vi "COM Stage Test Write.vi"() -> ()   [LabVIEW 2017]
panel:
  out "Numeric":i32
  in  "Position (mm)":dbl
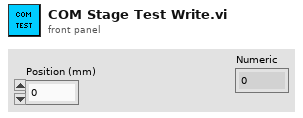
[diagram p1: front panel]
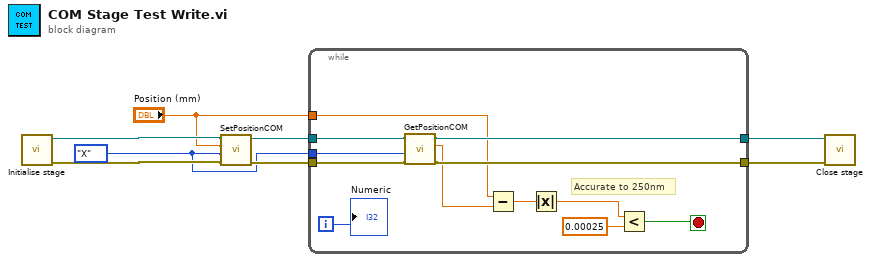
[diagram p0: block diagram]
diagram:
  w4 = enum16{"X", "Y", "Z"}."X" ("Axis")
  n1 = call "Initialise stage.vi"() -> ("error out"=w7:errorcluster, "Stage VISA reference"=w8:refnum<visa-resource-name>)  [unwired: 10 in]
  n2 = call "SetPositionCOM.vi"("error in"=w7, "Axis"=w4, "Position (mm)"="Position (mm)", "VISA resource name"=w8) -> ("error out"=w5:errorcluster, "VISA resource name out"=w6:refnum<visa-resource-name>)  [unwired: 6 in]
  n3 = while {
    tunnel: w6 -> [w17]
    tunnel: w5 -> [w15]
    tunnel: w4 -> [w16]
    tunnel: [w19] -> w3
    tunnel: [w18] -> w2
    tunnel: "Position (mm)" -> [w11]
    i -> [w20]
    stop <- w14 stop-if-true
    # "Accurate to 250nm"
    n4 = call "GetPositionCOM.vi"("error in"=w15, "Axis"=w16, "VISA resource name"=w17) -> ("error out"=w19:errorcluster, "Position (mm)"=w12:dbl, "VISA resource name out"=w18:refnum<visa-resource-name>)  [unwired: 6 in]
    n5 = Subtract(x=w11, y=w12) -> (x-y=w10:dbl)
    n6 = Absolute Value(x=w10) -> (abs(x)=w9:dbl)
    n7 = Less?(x=w9, y=0.00025) -> (x < y?=w14:bool)
    "Numeric" <- w20
  }
  n8 = call "Close stage.vi"("error in"=w3, "VISA resource name"=w2) -> ()  [unwired: 9 in, 1 out]
